vi "PH_ImageStatistician.ProcCases.vi"(0 "i ref in":refnum<vi>, 1 "selector":string, 2 "Data":T1, 3 "call cluster":T2={"Object"="", "Selector"="", "CallType"=enum."synchronous", "Async Object"="", "Async Selector"="", "Data Descriptor"="", "Data"=[], "Error #"=0, "Expire"=0}, 5 "error in (no error)":errorcluster) -> (14 "i ref out":refnum<vi>, 17 "answer cluster":T2={"Object"="", "Selector"="", "CallType"=enum."synchronous", "Async Object"="", "Async Selector"="", "Data Descriptor"="", "Data"=[], "Error #"=0, "Expire"=0}, 19 "error out":errorcluster)   [LabVIEW 2014, in "PH_ImageStatistician.lvlib"]
doc: "This method is called by a process from within the default case in the event loop. The methods of a class that are linked to events will be called from THIS method. Add your code here."
uses:
  PH_ImageStatistician.lvlib
  CSCore/CSSystem/CoreDefs/CoreDefs.call_type.ctl
  CSCore/BaseProcess/BaseProcess.descriptor string definition.ctl
  CSCore/CSSystem/CoreDefs/CoreDefs.rawDataType.ctl
  CSCore/CSSystem/CoreLib/CoreLib.byte array 2 short.vi
  CSCore/CSSystem/CoreLib/CoreLib.string 2 byte array.vi
  CSCore/CSSystem/CoreLib/CoreLib.lvlib
  CSCore/BaseProcess/BaseProcess.lvlib
  PH_PSDBWriter/PH_PSDBWriter.lvlib
  CSCore/CAEObj/CAEObj.lvlib
  PH_Common/PH_Common.lvlib
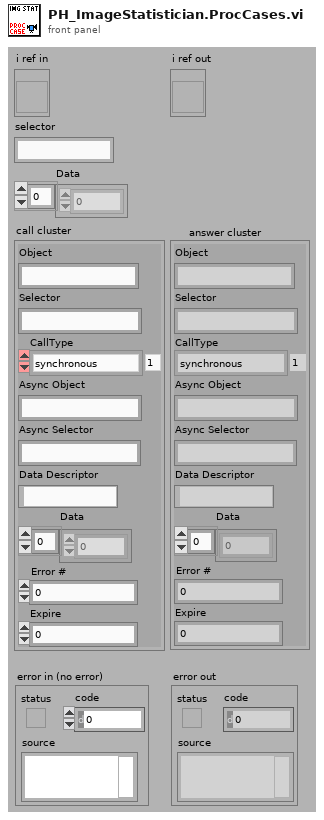
[diagram p1: front panel]
types:
  T1 = typedef "CoreDefs.rawDataType.ctl" = i8[]
  T2 = typedef "CoreDefs.call_type.ctl" = cluster{"Object":string, "Selector":string, "CallType":enum16{"simple", "synchronous", "asynchronous"}, "Async Object":string, "Async Selector":string, "Data Descriptor":T3, "Data":T1, "Error #":i32, "Expire":u32}
  T3 = typedef "BaseProcess.lvlib/BaseProcess.descriptor string definition.ctl" = string
  T4 = typedef "PH_ImageStatistician.lvlib/PH_ImageStatistician.i attribute.ctl" = cluster{"GUI Refs ":cluster{"Status":refnum<vi>, "Result Graph":refnum<vi>, "Mean Data 1":refnum<vi>, "Std Dev Data 1":refnum<vi>, "Mean Data 2":refnum<vi>, "Std Dev Data 2":refnum<vi>, "Mean Data 3":refnum<vi>, "Std Dev Data 3":refnum<vi>, "Dummy Mean":refnum<vi>, "Dummy Std Dev":refnum<vi>, "Export Data":refnum<vi>, "Data 1":refnum<vi>, "Data 2":refnum<vi>, "Data 3":refnum<vi>, "Stat or Trend":refnum<vi>, "Delete":refnum<vi>, "Operator":refnum<vi>, "Start":refnum<vi>}, "Operator":string, "Data":T5[], "Stat or Trend":bool, "Data 1":T6, "Data 2":T6, "Data 3":T6, "Start":bool, "Datasets strored":i32, "Dataarray Size":i32}
  T5 = typedef "PH_ImageStatistician.lvlib/PH_ImageStatistician.Statistician Data.ctl" = cluster{"Snapshot Time":dbl, "Maj FWHM":dbl, "Min FWHM":dbl, "Maj Fit Order":dbl, "Min Fit Order":dbl, "99% Diam Maj Trace":dbl, "99% Diam Min Trace":dbl, "Theta":dbl, "Delta":dbl, "Maj Diam":dbl, "Min Diam":dbl, "Azimuth Angle":dbl, "Azi Angle rel to major?":dbl, "Ellipticity":dbl, "CoG - X":dbl, "CoG - Y":dbl, "Energy":dbl, "Energy Cal - no mJ":dbl, "Lin Cal - no mm or mrad":dbl, "Lin Cal Factor":dbl}
  T6 = typedef "PH_ImageStatistician.lvlib/PH_ImageStatistician.select Data.ctl" = u16
  T7 = cluster{"[0]":dbl, "[1]":dbl, "[2]":dbl, "[3]":dbl, "[4]":dbl, "[5]":dbl, "[6]":dbl, "[7]":dbl, "[8]":dbl, "[9]":dbl, "[10]":dbl, "[11]":dbl, "[12]":dbl, "[13]":dbl, "[14]":dbl, "[15]":dbl, "[16]":dbl, "[17]":dbl, "[18]":dbl, "[19]":dbl}
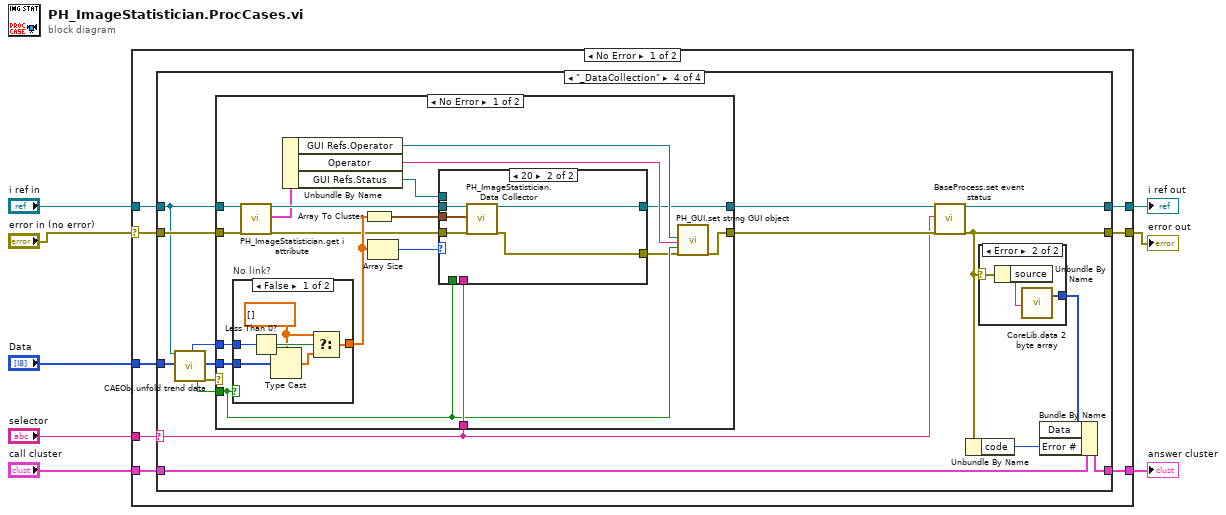
[diagram p0: block diagram]
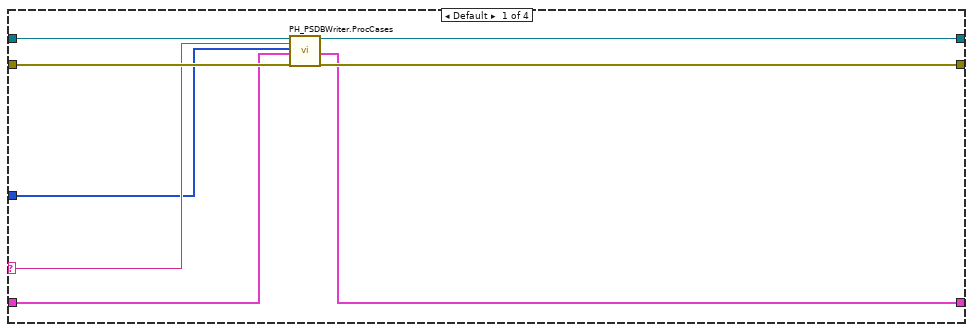
[diagram p2: hidden frame]
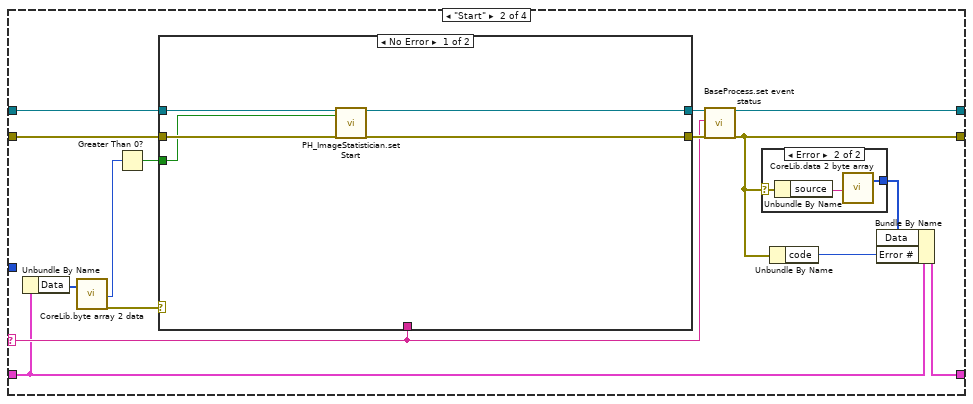
[diagram p3: hidden frame]
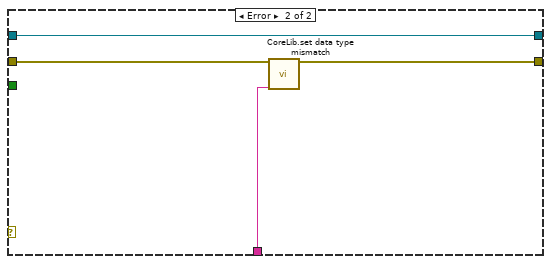
[diagram p5: hidden frame]
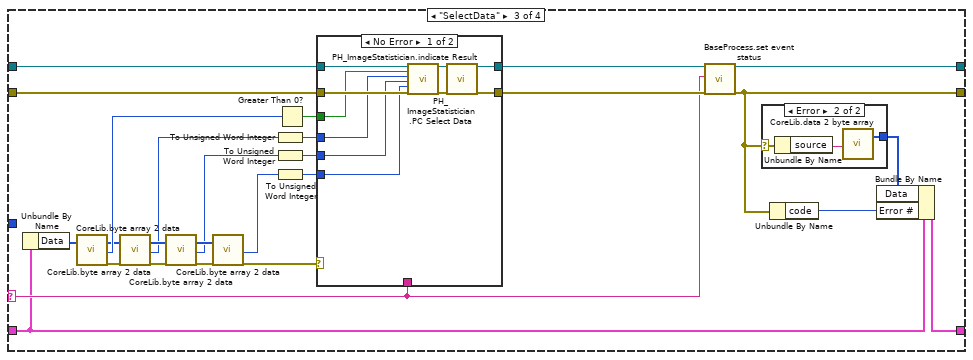
[diagram p6: hidden frame]
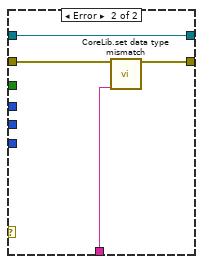
[diagram p8: hidden frame]
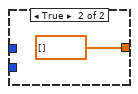
[diagram p10: hidden frame]
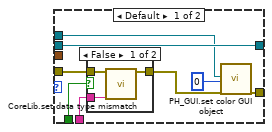
[diagram p11: hidden frame]
diagram:
  n1 = case shown="No Error" "error in (no error)" {
    selector: "error in (no error)" -> [w9 w162]
    tunnel: "selector" -> [w16 _]
    tunnel: [w15 w161] -> w7
    tunnel: "call cluster" -> [w14 w161]
    tunnel: "i ref in" -> [w13 w163]
    tunnel: [w12 w163] -> w5
    tunnel: [w11 w162] -> w4
    tunnel: "Data" -> [w10 _]
    frame No Error {
      n2 = case shown="\"_DataCollection\"" w16 {
        selector: w16 -> [w19 w28 w67 w104]
        tunnel: w13 -> [w18 w32 w71 w100]
        tunnel: [w24 w30 w69 w106] -> w12
        tunnel: w14 -> [w20 w27 w66 w103]
        tunnel: [w21 w26 w65 w102] -> w15
        tunnel: w9 -> [w23 w31 w70 w107]
        tunnel: [w22 w29 w68 w105] -> w11
        tunnel: w10 -> [w17 _ _ w101]
        frame Default {
          n3 = call "PH_PSDBWriter.ProcCases.vi"("i ref in"=w18, "selector"=w19, "Data"=w17, "call cluster"=w20, "error in"=w23) -> ("i ref out"=w24:refnum<vi>, "answer cluster"=w21:T2, "error out"=w22:errorcluster)  [unwired: 12 in]
        }
        frame "Start" {
          n4 = Unbundle By Name(w27) -> ("Data"=w35:T1)
          n5 = call-poly "CoreLib.byte array 2 data.vi"("byteArray"=w35) -> ("i16"=w36:i16, "error out"=w25:errorcluster)  [unwired: 16 in, 1 out]
          n6 = Greater Than 0?(x=w36) -> (x > 0?=w37:bool)
          n7 = case shown="No Error" w25 {
            tunnel: [w47 w51] -> w33
            tunnel: w32 -> [w46 w51]
            tunnel: w31 -> [w45 w50]
            tunnel: [w44 w49] -> w34
            tunnel: w28 -> [_ w48]
            tunnel: w37 -> [w43 _]
            frame No Error {
              n8 = call "PH_ImageStatistician.set Start.vi"("i ref in"=w46, "Start"=w43, "error in (no error)"=w45) -> ("i ref out"=w47:refnum<vi>, "error out"=w44:errorcluster)  [unwired: 15 in]
            }
            frame Error {
              n9 = call "CoreLib.set data type mismatch.vi"("error in (no error)"=w50, "error source"=w48) -> ("error out"=w49:errorcluster)  [unwired: 17 in]
            }
          }
          n10 = call "BaseProcess.set event status.vi"("i ref in"=w33, "EventStatus"=w28, "error in (no error)"=w34) -> ("i ref out"=w30:refnum<vi>, "error out"=w29:errorcluster)  [unwired: 14 in, 1 out]
          n11 = case shown="Error" w29 {
            selector: w29 -> [_ w42]
            tunnel: [_ w40] -> w39
            frame No Error {
            }
            frame Error {
              n12 = Unbundle By Name(w42) -> ("source"=w41:string)
              n13 = call-poly "CoreLib.data 2 byte array.vi"("string"=w41) -> ("byteArray out"=w40:T1)  [unwired: 18 in]
            }
          }
          n14 = Unbundle By Name(w29) -> ("code"=w38:i32)
          n15 = Bundle By Name(cluster=w27, "Data"=w39, "Error #"=w38) -> (w26:T2)
        }
        frame "SelectData" {
          n16 = Unbundle By Name(w66) -> ("Data"=w74:T1)
          n17 = call-poly "CoreLib.byte array 2 data.vi"("byteArray"=w74) -> ("byteArray out"=w60:T1, "i16"=w75:i16, "error out"=w64:errorcluster)  [unwired: 16 in]
          n18 = call-poly "CoreLib.byte array 2 data.vi"("byteArray"=w60, "error in (no error)"=w64) -> ("byteArray out"=w59:T1, "i16"=w57:i16, "error out"=w63:errorcluster)  [unwired: 15 in]
          n19 = call-poly "CoreLib.byte array 2 data.vi"("byteArray"=w59, "error in (no error)"=w63) -> ("byteArray out"=w58:T1, "i16"=w56:i16, "error out"=w62:errorcluster)  [unwired: 15 in]
          n20 = call-poly "CoreLib.byte array 2 data.vi"("byteArray"=w58, "error in (no error)"=w62) -> ("i16"=w55:i16, "error out"=w61:errorcluster)  [unwired: 15 in, 1 out]
          n21 = To Unsigned Word Integer(number=w57) -> (unsigned 16bit integer=w54:u16)
          n22 = To Unsigned Word Integer(number=w56) -> (unsigned 16bit integer=w53:u16)
          n23 = To Unsigned Word Integer(number=w55) -> (unsigned 16bit integer=w52:u16)
          n24 = Greater Than 0?(x=w75) -> (x > 0?=w76:bool)
          n25 = case shown="No Error" w61 {
            tunnel: [w84 w95] -> w72
            tunnel: w71 -> [w91 w95]
            tunnel: w70 -> [w90 w94]
            tunnel: [w82 w93] -> w73
            tunnel: w67 -> [_ w92]
            tunnel: w76 -> [w89 _]
            tunnel: w54 -> [w88 _]
            tunnel: w53 -> [w87 _]
            tunnel: w52 -> [w86 _]
            frame No Error {
              n26 = call "PH_ImageStatistician.PC Select Data.vi"("i ref in"=w91, "Stat or Trend"=w89, "Data 1"=w88, "Data 2"=w87, "Data 3"=w86, "error in (no error)"=w90) -> ("i ref out"=w85:refnum<vi>, "error out"=w83:errorcluster)  [unwired: 12 in]
              n27 = call "PH_ImageStatistician.indicate Result.vi"("i ref in"=w85, "error in (no error)"=w83) -> ("i ref out"=w84:refnum<vi>, "error out"=w82:errorcluster)  [unwired: 16 in]
            }
            frame Error {
              n28 = call "CoreLib.set data type mismatch.vi"("error in (no error)"=w94, "error source"=w92) -> ("error out"=w93:errorcluster)  [unwired: 17 in]
            }
          }
          n29 = call "BaseProcess.set event status.vi"("i ref in"=w72, "EventStatus"=w67, "error in (no error)"=w73) -> ("i ref out"=w69:refnum<vi>, "error out"=w68:errorcluster)  [unwired: 14 in, 1 out]
          n30 = case shown="Error" w68 {
            selector: w68 -> [_ w81]
            tunnel: [_ w79] -> w78
            frame No Error {
            }
            frame Error {
              n31 = Unbundle By Name(w81) -> ("source"=w80:string)
              n32 = call-poly "CoreLib.data 2 byte array.vi"("string"=w80) -> ("byteArray out"=w79:T1)  [unwired: 18 in]
            }
          }
          n33 = Unbundle By Name(w68) -> ("code"=w77:i32)
          n34 = Bundle By Name(cluster=w66, "Data"=w78, "Error #"=w77) -> (w65:T2)
        }
        frame "_DataCollection" {
          n35 = call "CAEObj.unfold trend data.vi"("i ref in"=w100, "raw trend data"=w101) -> ("quality"=w96:i32, "no link"=w98:bool, "data"=w97:i8[], "error out"=w99:errorcluster)  [unwired: 9 in, 5 out]
          n36 = case shown="No Error" w99 {
            tunnel: [w122 w160] -> w108
            tunnel: w100 -> [w119 w160]
            tunnel: w107 -> [w120 w159]
            tunnel: [w126 w158] -> w109
            tunnel: w104 -> [w130 w157]
            tunnel: w98 -> [w124 _]
            tunnel: w97 -> [w129 _]
            tunnel: w96 -> [w128 _]
            frame No Error {
              n37 = case "No link?" shown="False" w124 {
                tunnel: [w134 dbl[] []] -> w127
                tunnel: w128 -> [w138 _]
                tunnel: w129 -> [w137 _]
                frame False {
                  w133 = dbl[] []
                  n38 = Less Than 0?(x=w138) -> (x < 0?=w136:bool)
                  n39 = Type Cast(type=w133, x=w137) -> (*(type *) &x=w135:dbl[])
                  n40 = Select(t=w133, s=w136, f=w135) -> (s? t:f=w134:dbl[])
                }
                frame True {
                }
              }
              n41 = call "PH_ImageStatistician.get i attribute.vi"("i ref in"=w119, "error in (no error)"=w120) -> ("i ref out"=w118:refnum<vi>, "i attribute"=w116:T4, "error out"=w117:errorcluster)  [unwired: 15 in]
              n42 = Unbundle By Name(w116) -> ("GUI Refs.Operator"=w123:refnum<vi>, "Operator"=w125:string, "GUI Refs.Status"=w115:refnum<vi>)
              n43 = Array To Cluster(array=w127) -> (cluster=w132:T7)
              n44 = Array Size(array=w127) -> (size(s)=w131:i32)
              n45 = case shown="20" w131 {
                tunnel: [w146 w156] -> w122
                tunnel: [w142 w155] -> w121
                tunnel: w118 -> [w146 w154]
                tunnel: w117 -> [w147 w153]
                tunnel: w132 -> [_ w152]
                tunnel: w130 -> [w145 _]
                tunnel: w124 -> [w144 _]
                tunnel: w115 -> [w140 _]
                frame Default {
                  n46 = case shown="False" w144 {
                    tunnel: w147 -> [w150 w151]
                    tunnel: [w149 w151] -> w143
                    tunnel: w145 -> [w148 _]
                    frame False {
                      n47 = call "CoreLib.set data type mismatch.vi"("error in (no error)"=w150, "error source"=w148) -> ("error out"=w149:errorcluster)  [unwired: 17 in]
                    }
                    frame True {
                    }
                  }
                  n48 = call "PH_GUI.set color GUI object.vi"("GUI object Ref"=w140, "State"=0, "error in (no error)"=w143) -> ("error out"=w142:errorcluster)  [unwired: 16 in]
                }
                frame 20 {
                  n49 = call "PH_ImageStatistician.Data Collector.vi"("i ref in"=w154, "Img Op Dataset"=w152, "error in (no error)"=w153) -> ("i ref out"=w156:refnum<vi>, "error out"=w155:errorcluster)  [unwired: 15 in]
                }
              }
              n50 = call "PH_GUI.set string GUI object.vi"("GUI object Ref"=w123, "Text"=w125, "Blinking? (false)"=w124, "error in"=w121) -> ("error out"=w126:errorcluster)  [unwired: 15 in]
            }
            frame Error {
              n51 = call "CoreLib.set data type mismatch.vi"("error in (no error)"=w159, "error source"=w157) -> ("error out"=w158:errorcluster)  [unwired: 17 in]
            }
          }
          n52 = call "BaseProcess.set event status.vi"("i ref in"=w108, "EventStatus"=w104, "error in (no error)"=w109) -> ("i ref out"=w106:refnum<vi>, "error out"=w105:errorcluster)  [unwired: 14 in, 1 out]
          n53 = Unbundle By Name(w105) -> ("code"=w110:i32)
          n54 = case shown="Error" w105 {
            selector: w105 -> [_ w114]
            tunnel: [_ w112] -> w111
            frame No Error {
            }
            frame Error {
              n55 = Unbundle By Name(w114) -> ("source"=w113:string)
              n56 = call-poly "CoreLib.data 2 byte array.vi"("string"=w113) -> ("byteArray out"=w112:T1)  [unwired: 18 in]
            }
          }
          n57 = Bundle By Name(cluster=w103, "Data"=w111, "Error #"=w110) -> (w102:T2)
        }
      }
    }
    frame Error {
    }
  }
  "answer cluster" <- w7
  "i ref out" <- w5
  "error out" <- w4
